vi "_dataFlag.vi"(8 "error in (no error)":errorcluster, 11 "DB Ref":T1) -> (0 "error in (no error) (dup)":errorcluster, 2 "DataChangeFlag":i64, 3 "DB Ref (dup)":T1)   [LabVIEW 2014, in "TagDB(dev).lvlib"]
uses:
  TagDB(dev).lvlib
  tagDB_Def.ctl
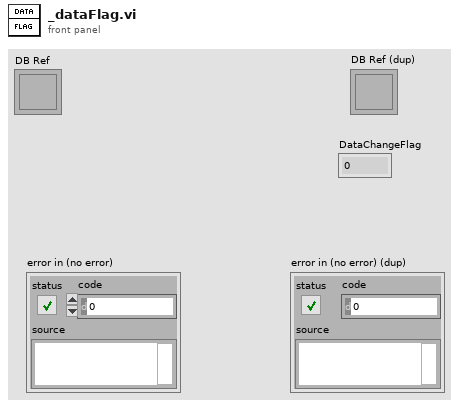
[diagram p1: front panel]
types:
  T1 = typedef "TagDB(dev).lvlib/tagDB_Def.ctl" = refnum<k1>
  T2 = typedef "TagDB(dev).lvlib/_DEF-DATA.ctl" = cluster{"data hashmap":variant, "DataChangeFlag":i64, "ItemChangeFlag":i64, "name":string, "Tag Adding Lock?":bool}
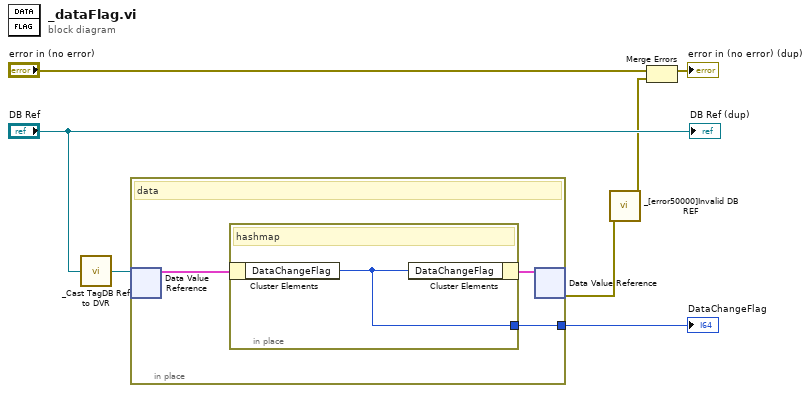
[diagram p0: block diagram]
diagram:
  n1 = call "_Cast TagDB Ref to DVR.vi"("TagDB"="DB Ref") -> ("DVR"=w5:refnum<data-value>)  [unwired: 4 in]
  n2 = in-place {
    in-place-border: [w8] -> w3
    # "data"
    n3 = in-place-dvr #1(w5) -> (w10:T2)  [unwired: 1 out]
    n4 = in-place {
      in-place-border: [w11] -> w8
      # "hashmap"
      n5 = in-place-cluster #2(w10) -> ("DataChangeFlag"=w11:i64)
      n6 = in-place-cluster #2("DataChangeFlag"=w11) -> (w9:T2)
    }
    n7 = in-place-dvr #1(w9) -> (w4:errorcluster)  [unwired: 1 out]
  }
  "DataChangeFlag" <- w3
  n8 = call "_[error50000]Invalid DB REF.vi"("error in (no error)"=w4) -> ("error out"=w1:errorcluster)  [unwired: 10 in]
  n9 = Merge Errors("error in (no error)", w1) -> (→"error in (no error) (dup)":errorcluster)
  "DB Ref (dup)" <- "DB Ref"
